vi "Make Receiver.vi"(8 "error in (no error)":errorcluster, 11 "Abstract Message Scripter in":refnum<class "Abstract Message Scripter.lvclass">) -> (0 "error out":errorcluster, 3 "Abstract Message Scripter out":refnum<class "Abstract Message Scripter.lvclass">)   [LabVIEW 2020, in "Message Maker.lvlib" / "Abstract Message Scripter.lvclass"]
uses:
  Abstract Message Scripter.lvclass
  Message Maker.lvlib
  Message Scripter/Message Scripter.lvclass
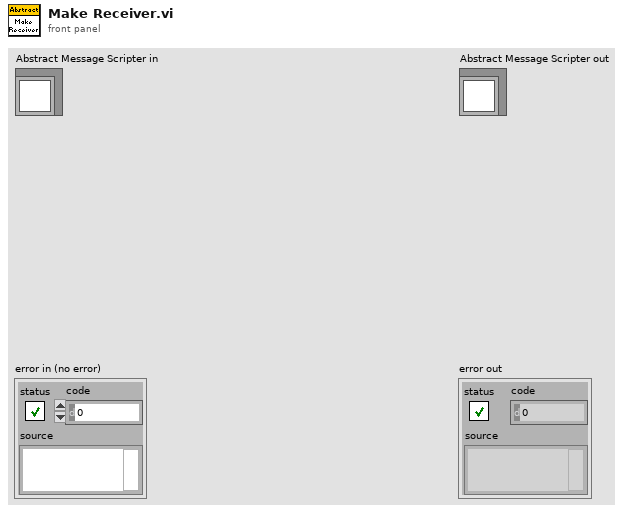
[diagram p1: front panel]
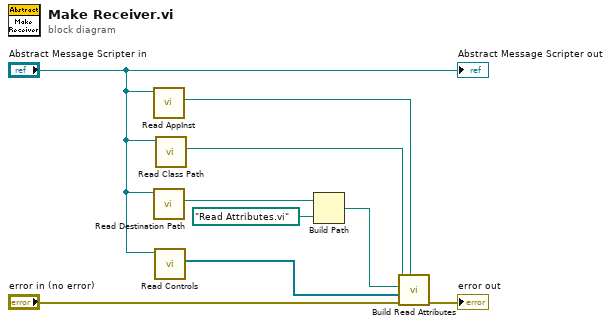
[diagram p0: block diagram]
diagram:
  n1 = call "Read AppInst.vi"("Message Maker in"="Abstract Message Scripter in") -> ("AppInst"=w6:refnum<vi>)  [unwired: 10 in]
  n2 = call "Read Destination Path.vi"("Message Scripter in"="Abstract Message Scripter in") -> ("Destination Path"=w7:path)  [unwired: 10 in]
  n3 = call "Read Controls.vi"("Message Scripter in"="Abstract Message Scripter in") -> ("Controls[]"=w3:refnum<vi>[])  [unwired: 9 in, 1 out]
  n4 = call "Read Class Path.vi"("Message Scripter in"="Abstract Message Scripter in") -> ("Class Path"=w1:path)  [unwired: 10 in]
  n5 = Build Path(base path=w7, name or relative path=path "Read Attributes.vi") -> (appended path=w8:path)
  n6 = call "Build Read Attributes.vi"("AppInst"=w6, "error in (no error)"="error in (no error)", "Controls"=w3, "Read Attributes path"=w8, "Class Library"=w1) -> ("error out"=→"error out":errorcluster)  [unwired: 6 in]
  "Abstract Message Scripter out" <- "Abstract Message Scripter in"
